vi "test_easy_linear_interpl.vi"() -> ()   [LabVIEW 2009]
doc: "Copyright (C) 2009, Stepan A. Baranov\nweb: http://www.OCTLab.org/\nemail: stepan@baranov.su"
uses:
  OCTLib.dll
  <vilib>/gmath/NI_Gmath.lvlib
panel:
  out "RSM_STAT final 2D array":dbl[](array[numeric])
  out "error out":errorcluster
  out "data Graph":dbl[][](graph)
  out "wavelengths Graph":dbl[][](graph)
  out "LabView final 2D array":dbl[](array[numeric])
  out "initial 2D array":dbl[](array[numeric])
  in  "stop":bool
  in  "index (row)":i32=1
  in  "Y":i32=9
  in  "X":i32=800
  in  "End wavelength":dbl=890.0
  in  "Start wavelength":dbl=800.0
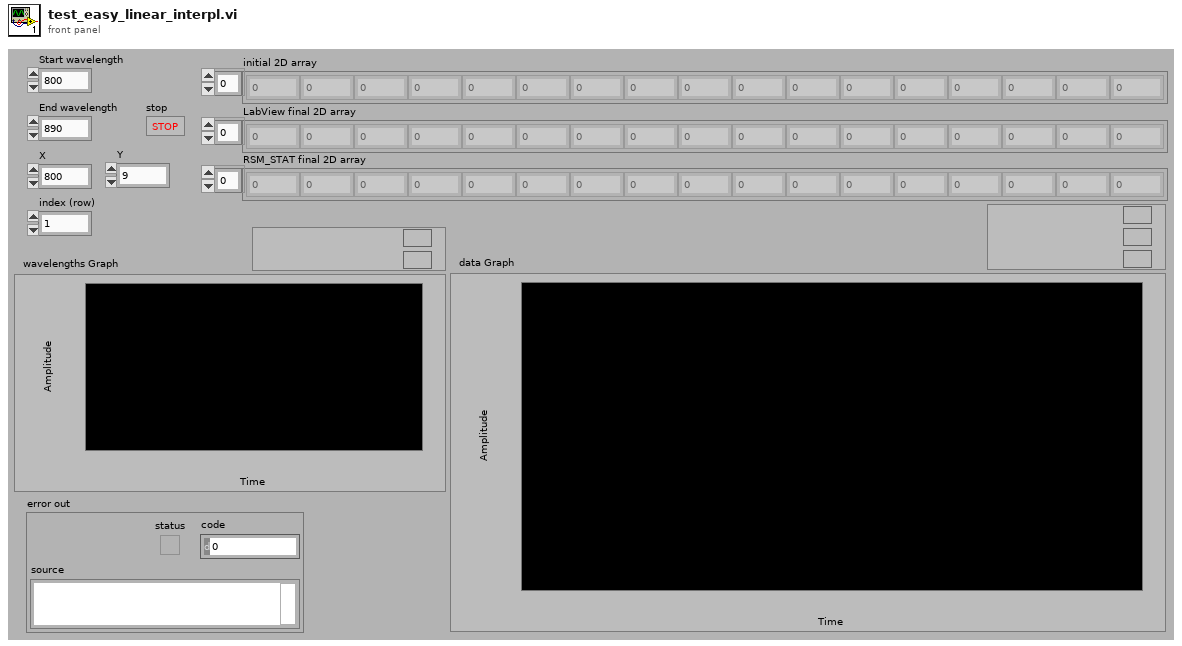
[diagram p1: front panel]
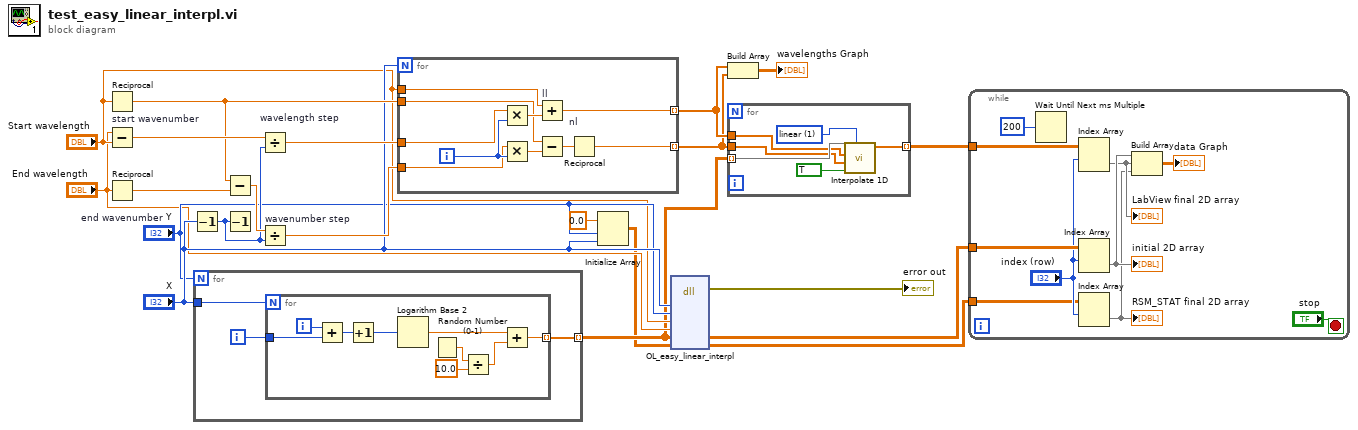
[diagram p0: block diagram]
diagram:
  n1 = Reciprocal "start wavenumber"(x="Start wavelength") -> (1/x=w15:dbl)
  n2 = Subtract(x="End wavelength", y="Start wavelength") -> (x-y=w21:dbl)
  n3 = Reciprocal "end wavenumber"(x="End wavelength") -> (1/x=w20:dbl)
  n4 = Decrement(x="X") -> (x-1=w18:i32)
  n5 = for {
    N: "Y" -> [_]
    tunnel: [w24] -> w8 mode=indexing
    tunnel: "X" -> [w23]
    i -> [w22]
    n6 = for {
      N: w23 -> [_]
      tunnel: [w32] -> w24 mode=indexing
      tunnel: w22 -> [w33]
      i -> [w31]
      n7 = Add(x=w31, y=w33) -> (x+y=w30:i32)
      n8 = Increment(x=w30) -> (x+1=w29:i32)
      n9 = Logarithm Base 2(1:w29) -> (0:w28:dbl)
      n10 = Random Number (0-1)() -> (number: 0 to 1=w27:dbl)
      n11 = Divide(x=w27, y=10.0) -> (x/y=w25:dbl)
      n12 = Add(x=w28, y=w25) -> (x+y=w32:dbl)
    }
  }
  n13 = Subtract(x=w15, y=w20) -> (x-y=w19:dbl)
  n14 = Decrement(x=w18) -> ()  [unwired: 1 out]
  n15 = Divide "wavelength step"(x=w21, y=w18) -> (x/y=w17:dbl)
  n16 = Divide "wavenumber step"(x=w19, y=w18) -> (x/y=w16:dbl)
  n17 = for {
    N: "X" -> [_]
    tunnel: w17 -> [w43]
    tunnel: "Start wavelength" -> [w41]
    tunnel: [w40] -> w4 mode=indexing
    tunnel: w16 -> [w38]
    tunnel: w15 -> [w35]
    tunnel: [w34] -> w3 mode=indexing
    i -> [w39]
    n18 = Multiply(x=w43, y=w39) -> (x*y=w42:dbl)
    n19 = Multiply(x=w38, y=w39) -> (x*y=w36:dbl)
    n20 = Add "ll"(x=w41, y=w42) -> (x+y=w40:dbl)
    n21 = Subtract(x=w35, y=w36) -> (x-y=w37:dbl)
    n22 = Reciprocal "nl"(x=w37) -> (1/x=w34:dbl)
  }
  n23 = Initialize Array(0.0 ("element"), "Y", "X") -> (w7:dbl[][])
  n24 = dll-call lib="OCTLib.dll" fn="OL_easy_linear_interpl"("width"="X", "height"="Y", "start_wavelength"="Start wavelength", "end_wavelength"="End wavelength", "in"=w8, "out"=w7) -> (error out=→"error out":errorcluster, "in"=w1:dbl[][], "out"=w6:dbl[][])  [unwired: 8 in, 1 out]
  n25 = Build Array(w4, w3) -> (→"wavelengths Graph":dbl[][])
  n26 = for {
    tunnel: w8 -> [w47] mode=indexing
    tunnel: w4 -> [w46]
    tunnel: w3 -> [w45]
    tunnel: [w44] -> w2 mode=indexing
    w48 = 1 items=["nearest", "linear", "spline", "cubic Hermite", "Lagrange"] ("method")
    n27 = call <vilib>:"Interpolate 1D.vi"("method"=w48, "X is monotonic"=TRUE, "xi"=w45, "X"=w46, "Y"=w47) -> ("yi"=w44:dbl[])  [unwired: 4 in, 2 out]
  }
  n28 = while {
    tunnel: w2 -> [w59]
    tunnel: w1 -> [w56]
    tunnel: w6 -> [w54]
    stop <- "stop" stop-if-true
    n29 = Wait Until Next ms Multiple(millisecond multiple=u32 200) -> ()  [unwired: 1 out]
    n30 = Index Array(array=w59, index (row)="index (row)") -> (element=w52:dbl[])  [unwired: 1 in]
    "LabView final 2D array" <- w52
    n31 = Index Array(array=w56, index (row)="index (row)") -> (element=w53:dbl[])  [unwired: 1 in]
    "initial 2D array" <- w53
    n32 = Index Array(array=w54, index (row)="index (row)") -> (element=w51:dbl[])  [unwired: 1 in]
    "RSM_STAT final 2D array" <- w51
    n33 = Build Array(w53, w52, w51) -> (→"data Graph":dbl[][])
  }
